vi "Insert Menu Panels.vi"(8 "错误输入":errorcluster, 10 "Static VI*":refnum<vi>, 11 "Node*":refnum<data-value>) -> (0 "error out":errorcluster)   [LabVIEW 2016, in "PCM PanelSplit.lvclass"]
uses:
  PCM PanelSplit.lvclass
  PanelSplitToolkit/PanelObject/PanelObject.lvclass
  PanelSplitToolkit/PanelDataNode/PanelDataNode.lvclass
  C:/Users/CL/Desktop/ZcDAQprj0811/ZcDAQprj/Modules/DAQ-Display/PanelSplitToolkit/PanelLinkNode/PanelLinkNode.lvclass
  PanelSplitToolkit/PanelLinkNode/PanelLinkNode.lvclass/PanelLinkNode.ctl
  PanelSplitToolkit/PanelDataNode/PanelDataNode.lvclass/PanelDataNode.ctl
  PanelSplitToolkit/PanelLinkNode/PanelLinkNode.lvclass
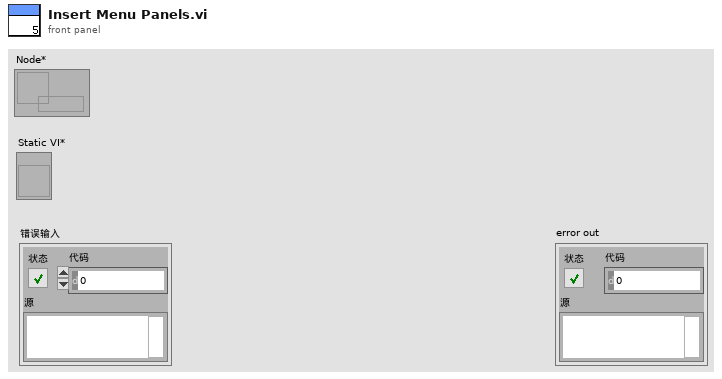
[diagram p1: front panel]
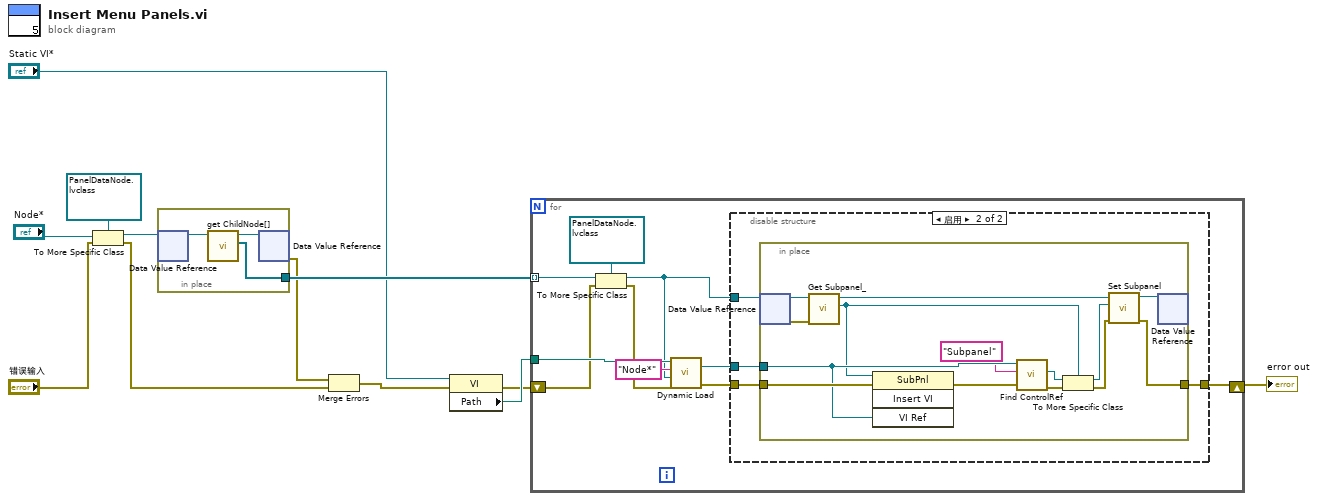
[diagram p0: block diagram]
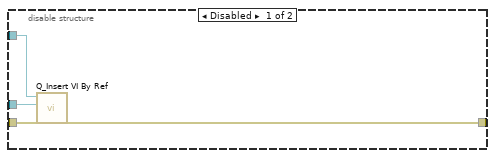
[diagram p2: hidden frame]
diagram:
  n1 = To More Specific Class(target class=refnum<data-value> refnum ("ChildNode*"), reference="Node*", error in="错误输入") -> (specific class reference=w9:refnum<data-value>, error out=w4:errorcluster)
  n2 = in-place {
    in-place-border: [w13] -> w8
    n3 = in-place-dvr #1(w9) -> (w15:refnum<class "PanelDataNode.lvclass">)  [unwired: 1 out]
    n4 = call "get ChildNode[].vi"("PanelLinkNode输入"=w15) -> ("ChildNode*[]"=w13:refnum<data-value>[], "PanelLinkNode输出"=w14:refnum<class "PanelDataNode.lvclass">)  [unwired: 8 in, 1 out]
    n5 = in-place-dvr #1(w14) -> (w5:errorcluster)  [unwired: 1 out]
  }
  n6 = Merge Errors(w5, w4) -> (w3:errorcluster)
  n7 = property class="VI"(reference="Static VI*", error in=w3) -> (error out=w11:errorcluster, "Path"=w12:path)  [unwired: 1 out]
  n8 = for {
    tunnel: w12 -> [w25]
    tunnel: w8 -> [w18] mode=indexing
    shift-right: [w23] -> w6
    shift-left: w11 -> [w20]
    n9 = To More Specific Class(target class=refnum<data-value> refnum ("ChildNode*"), reference=w18, error in=w20) -> (specific class reference=w16:refnum<data-value>, error out=w19:errorcluster)
    n10 = call "Dynamic Load.vi"("error in"=w19, "CtrlValue"=w16, "CtrlName"="Node*", "Vi Path"=w25) -> ("错误输出"=w24:errorcluster, "vi reference"=w22:refnum<vi>)  [unwired: 6 in]
    n11 = disable-structure shown="启用" {
      disable-tunnel: w24 -> [w29 w31]
      disable-tunnel: [w28 w30] -> w23
      disable-tunnel: w22 -> [w27 w32]
      disable-tunnel: w16 -> [w26 w33]
      frame Disabled {
        n12 = call "Q_Insert VI By Ref.vi"("error in"=w29, "Dynamic VI*"=w27, "ChildNode*"=w26) -> ("error out"=w28:errorcluster)  [unwired: 8 in]
      }
      frame Enabled {
        n13 = in-place {
          in-place-border: w32 -> [w44]
          in-place-border: w31 -> [w45]
          in-place-border: [w35] -> w30
          n14 = in-place-dvr #2(w33) -> (w47:refnum<class "PanelDataNode.lvclass">, w46:errorcluster)
          n15 = call-dynamic "Get Subpanel_.vi"("error in (no error)"=w46, "PanelDataNode输入"=w47) -> ("Subpanel*"=w38:refnum<vi>, "PanelDataNode输出"=w42:refnum<class "PanelDataNode.lvclass">)  [unwired: 7 in, 1 out]
          n16 = invoke class="SubPnl" method="Insert VI"(reference=w38, error in=w45, "VI Ref"=w44) -> (error out=w43:errorcluster)  [unwired: 1 in, 3 out]
          n17 = call "Find ControlRef.vi"("error in (no error)"=w43, "control name"="Subpanel", "vi*"=w44) -> ("error out"=w40:errorcluster, "ctrl*"=w39:refnum<vi>)  [unwired: 6 in, 1 out]
          n18 = To More Specific Class(target class=w38, reference=w39, error in=w40) -> (specific class reference=w37:refnum<vi>, error out=w36:errorcluster)
          n19 = call "Set Subpanel.vi"("error in (no error)"=w36, "Subpanel*"=w37, "PanelDataNode输入"=w42) -> ("error out"=w35:errorcluster, "PanelDataNode输出"=w34:refnum<class "PanelDataNode.lvclass">)  [unwired: 7 in]
          n20 = in-place-dvr #2(w34) -> ()  [unwired: 2 out]
        }
      }
    }
  }
  "error out" <- w6
